vi "TLPM Get Resource Information.vi"(8 "error in (no error)":errorcluster {"code" format="%.0x"}, 10 "Index (0)":u32, 11 "instrument handle":refnum<visa-resource-name>) -> (0 "error out":errorcluster {"code" format="%.0x"}, 1 "Serial Number":string, 2 "Model Name":string, 3 "instrument handle out":refnum<visa-resource-name>, 4 "Manufacturer":string, 5 "Device Available":bool)   [LabVIEW 2019]
doc: "This VI gets information about a connected resource.\n\nNotes:\n(1) The data provided by this VI was updated at the last call of <Find Resources>."
uses:
  TLPM_32.dll
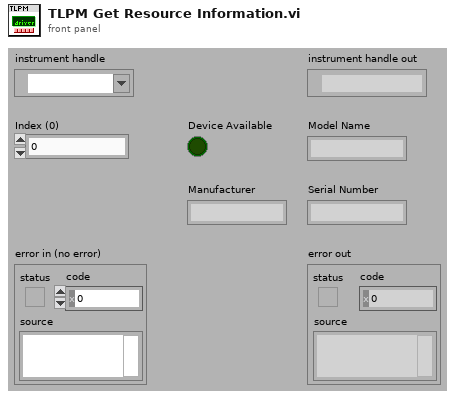
[diagram p1: front panel]
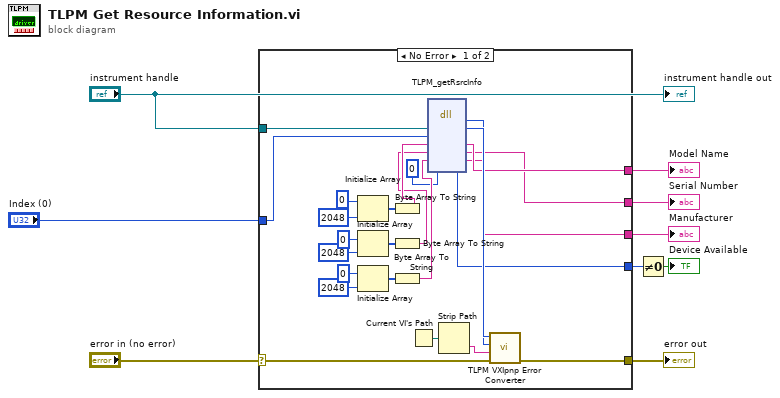
[diagram p0: block diagram]
diagram:
  n1 = case shown="No Error" "error in (no error)" {
    selector: "error in (no error)" -> [w29 w35]
    tunnel: [w28 w35] -> w9
    tunnel: "instrument handle" -> [w33 _]
    tunnel: "Index (0)" -> [w27 _]
    tunnel: [w22 _] -> w5
    tunnel: [w17 _] -> w4
    tunnel: [w12 _] -> w3
    tunnel: [w10 _] -> w1
    frame No Error {
      n2 = Initialize Array(u8 0 ("element"), 2048 ("dimension size")) -> (w25:u8[])
      n3 = Initialize Array(u8 0 ("element"), 2048 ("dimension size")) -> (w20:u8[])
      n4 = Initialize Array(u8 0 ("element"), 2048 ("dimension size")) -> (w15:u8[])
      n5 = Byte Array To String(unsigned byte array=w25) -> (string=w26:string)
      n6 = Byte Array To String(unsigned byte array=w20) -> (string=w21:string)
      n7 = Byte Array To String(unsigned byte array=w15) -> (string=w16:string)
      n8 = Current VI's Path() -> (path=w34:path)
      n9 = dll-call lib="TLPM_32.dll" fn="TLPM_getRsrcInfo"("Instrument Handle"=w33, "Index"=w27, "Model Name"=w26, "Serial Number"=w21, "Manufacturer"=w16, "Device Available"=i16 0) -> (w31:i32, "Instrument Handle"=w32:u32, "Model Name"=w22:string, "Serial Number"=w17:string, "Manufacturer"=w12:string, "Device Available"=w10:i16)  [unwired: 4 in, 2 out]
      n10 = Strip Path(path=w34) -> (name=w30:string)  [unwired: 1 out]
      n11 = call <userlib>:"TLPM VXIpnp Error Converter.vi"("error in (no error)"=w29, "Name Of VI (\"\")"=w30, "CVI Error Code (0)"=w31, "instrument handle"=w32) -> ("error out"=w28:errorcluster)  [unwired: 6 in, 1 out]
    }
    frame Error {
    }
  }
  "error out" <- w9
  "Model Name" <- w5
  "Serial Number" <- w4
  "Manufacturer" <- w3
  n12 = Not Equal To 0?(x=w1) -> (x != 0?=→"Device Available":bool)
  "instrument handle out" <- "instrument handle"
